vi "Get CUR wrapper.vi"(8 "error in (no error)":errorcluster caption="错误输入（无错误）", 10 "dwCanNodeId":u32, 11 "dwDevIndex":u32) -> (0 "error out":errorcluster caption="错误输出", 1 "current":dbl, 3 "function return":u32)   [LabVIEW 2016, in "UISimCanFunc_wrapper.lvlib"]
doc: "_declspec (dllexport) DWORD GetCUR_wrapper(DWORD dwDevIndex, DWORD dwCanNodeId, P_BASIC_ACK_OBJ pACKInfo);"
uses:
  <userlib>/UISimCanFunc_wrapper/UISimCanFunc_wrapper.lvlib
  <userlib>/UISimCanFunc_wrapper/UISimCanFunc_wrapper.dll
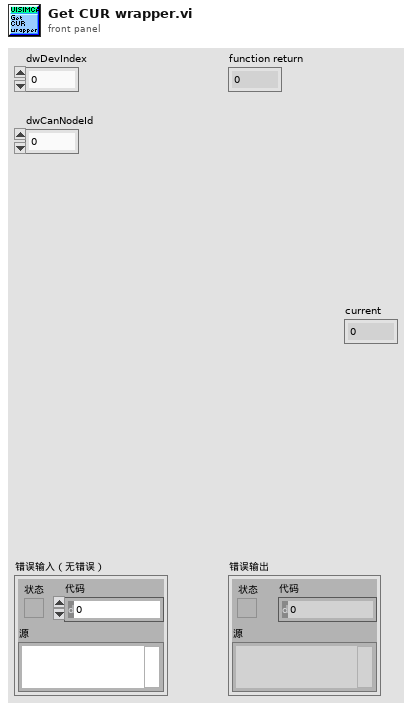
[diagram p1: front panel]
types:
  T1 = cluster{"uiReserv":u32, "bENA":i32, "bDIR":i32, "bACR":i32, "uiMCS":u32, "uiCUR":u32, "uiSPD":u32, "uiSTP":u32}
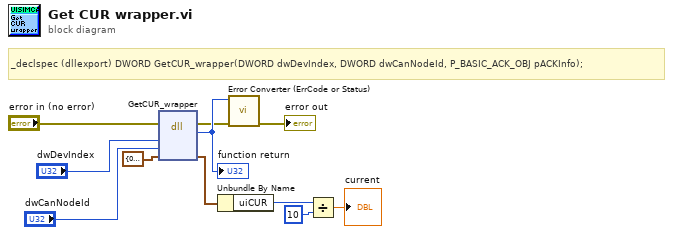
[diagram p0: block diagram]
diagram:
  # "_declspec (dllexport) DWORD GetCUR_wrapper(DWORD dwDevIndex, DWORD dwCanNodeId, P_BASIC_ACK_OBJ pACKInfo);"
  n1 = dll-call lib="C:/Program Files (x86)/National Instruments/LabVIEW 2016/user.lib/UISimCanFunc_wrapper/UISimCanFunc_wrapper.*" fn="GetCUR_wrapper"(error in="error in (no error)", "dwDevIndex"="dwDevIndex", "dwCanNodeId"="dwCanNodeId", "pACKInfo"=T1 {"uiReserv"=0, "bENA"=0, "bDIR"=0, "bACR"=0, "uiMCS"=0, "uiCUR"=0, "uiSPD"=0, "uiSTP"=0}) -> (error out=w6:errorcluster, w11:u32, "pACKInfo"=w4:T1)  [unwired: 4 in, 1 out]
  "function return" <- w11
  n2 = Unbundle By Name(w4) -> ("uiCUR"=w3:u32)
  n3 = call <userlib>:"Error Converter (ErrCode or Status).vi"("error in (no error)"=w6, "error code"=w11) -> ("error out"=→"error out":errorcluster)  [unwired: 9 in]
  n4 = Divide(x=w3, y=10) -> (x/y=→"current":dbl)
